vi "Calcul Aire Autocco.vi"(7 "Spectre-BKG":dbl[](array[numeric]), 8 "error in (no error)":errorcluster caption="entrée d'erreur (pas d'erreur)", 9 "PosX.Curs-1":dbl, 10 "PosX.Curs-0":dbl, 11 "UI SA en entrée":refnum<class "UI SmarAct.lvclass">) -> (0 "error out":errorcluster caption="sortie d'erreur", 2 "Aire Autocco":dbl, 3 "UI SA en sortie":refnum<class "UI SmarAct.lvclass">)   [LabVIEW 2024, in "UI SmarAct.lvclass"]
uses:
  UI SmarAct.lvclass
  UI SmarAct.lvclass/UI SmarAct.ctl
  <vilib>/Analysis/8numeric.llb/1D Numeric Integration.vi
  <vilib>/Analysis/NI_AALPro.lvlib
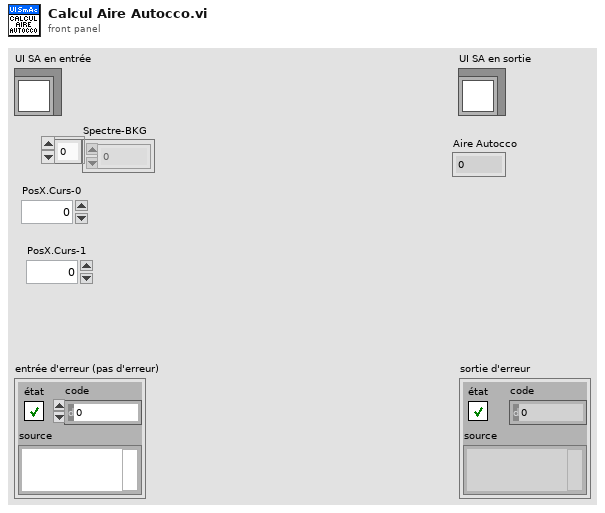
[diagram p1: front panel]
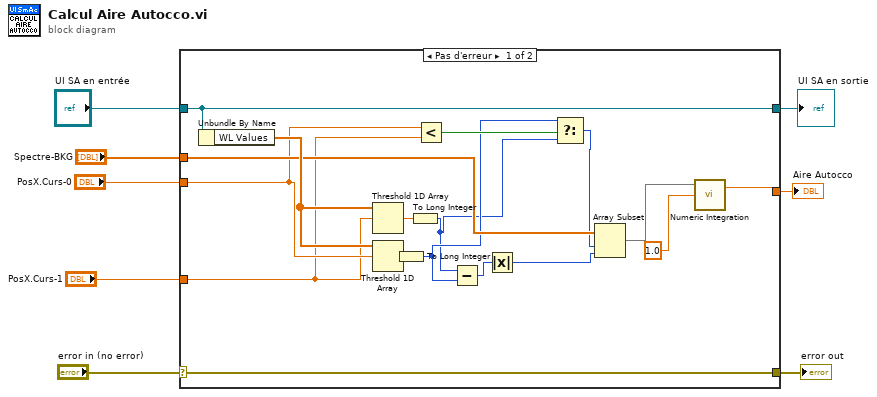
[diagram p0: block diagram]
diagram:
  n1 = case shown="Pas d'erreur" "error in (no error)" {
    selector: "error in (no error)" -> [w25 w27]
    tunnel: [w25 w27] -> w7
    tunnel: [w19 w26] -> w5
    tunnel: "UI SA en entrée" -> [w19 w26]
    tunnel: "PosX.Curs-0" -> [w14 _]
    tunnel: "PosX.Curs-1" -> [w13 _]
    tunnel: "Spectre-BKG" -> [w17 _]
    tunnel: [w16 _] -> w1
    frame No Error {
      n2 = Unbundle By Name(w19) -> ("WL Values"=w18:dbl[])
      n3 = Threshold 1D Array(2:w13, 3:w18) -> (0:w24:dbl)  [unwired: 1 in]
      n4 = Threshold 1D Array(2:w14, 3:w18) -> (0:w22:dbl)  [unwired: 1 in]
      n5 = To Long Integer(number=w22) -> (32bit integer=w11:i32)
      n6 = To Long Integer(number=w24) -> (32bit integer=w10:i32)
      n7 = Less?(x=w14, y=w13) -> (x < y?=w15:bool)
      n8 = Subtract(x=w10, y=w11) -> (x-y=w23:i32)
      n9 = Absolute Value(x=w23) -> (abs(x)=w12:i32)
      n10 = Select(t=w11, s=w15, f=w10) -> (s? t:f=w9:i32)
      n11 = Array Subset(array=w17, index=w9, length=w12) -> (w21:dbl[])
      n12 = call-poly <vilib>:"Numeric Integration.vi"("dt"=1.0, "Input Array"=w21) -> ("result"=w16:dbl)  [unwired: 1 in, 1 out]
    }
    frame Error {
    }
  }
  "error out" <- w7
  "UI SA en sortie" <- w5
  "Aire Autocco" <- w1
